vi "GetProbePlanCoordinates.vi"(8 "Use index as X coord":bool=TRUE, 9 "Probe Card Channels":i32=1) -> (0 "file path":string, 2 "OK?":bool, 3 "Array":T1(array[cluster]))   [LabVIEW 2018] (continued)
  out "String":string="There\tmust\tbe\tat\tleast\tone\tregion\nRegion=Segment\t3T\nLabel=Strip\t1\tX=-1082.31\ty=-40425.51 \nLabel=Strip\t2\tX=-725.71\ty=-40380.45 \nLabel=Strip\t3\tX=-1066.76\ty=-40277.87 \nLabel=Strip\t4\tX=-710.17\ty=-40232.68 \nLabel=Strip\t5\tX=-1051.26\ty=-40130.23 \nLabel=Strip\t6\tX=-694.70\ty=-40084.90 \nLabel=Strip\t7\tX=-1035.82\ty=-39982.58 \nLabel=Strip\t8\tX=-679.28\ty=-39937.11 \nLabel=Strip\t9\tX=-1020.44\ty=-39834.92 \nLabel=Strip\t10\tX=-663.91\ty=-39789.32 \nLabel=Strip\t11\tX=-1005.12\ty=-39687.26 \nLabel=Strip\t12\tX=-648.61\ty=-39641.51 \nLabel=Strip\t13\tX=-989.85\ty=-39539.59 \nLabel=Strip\t14\tX=-633.36\ty=-39493.70 \nLabel=Strip\t15\tX=-974.64\ty=-39391.91 \nLabel=Strip\t16\tX=-618.16\ty=-39345.89 \nLabel=Strip\t17\tX=-959.49\ty=-39244.23 \nLabel=Strip\t18\tX=-603.03\ty=-39198.06 \nLabel=Strip\t19\tX=-944.39\ty=-39096.54 \nLabel=Strip\t20\tX=-587.95\ty=-39050.23 \nLabel=Strip\t21\tX=-929.35\ty=-38948.84 \nLabel=Strip\t22\tX=-572.93\ty=-38902.40 \nLabel=Strip\t23\tX=-914.37\ty=-38801.13 \nLabel=Strip\t24\tX=-557.96\ty=-38754.55 \nLabel=Strip\t25\tX=-899.44\ty=-38653.42 \nLabel=Strip\t26\tX=-543.05\ty=-38606.70 \nLabel=Strip\t27\tX=-884.57\ty=-38505.70 \nLabel=Strip\t28\tX=-528.20\ty=-38458.84 \nLabel=Strip\t29\tX=-869.76\ty=-38357.97 \nLabel=Strip\t30\tX=-513.41\ty=-38310.98 \nLabel=Strip\t31\tX=-855.00\ty=-38210.23 \nLabel=Strip\t32\tX=-498.67\ty=-38163.10 \nLabel=Strip\t33\tX=-840.30\ty=-38062.49 \nLabel=Strip\t34\tX=-483.98\ty=-38015.22 \nLabel=Strip\t35\tX=-825.66\ty=-37914.74 \nLabel=Strip\t36\tX=-469.36\ty=-37867.34 \nLabel=Strip\t37\tX=-811.07\ty=-37766.99 \nLabel=Strip\t38\tX=-454.79\ty=-37719.44 \nLabel=Strip\t39\tX=-796.54\ty=-37619.23 \nLabel=Strip\t40\tX=-440.28\ty=-37571.54 \nLabel=Strip\t41\tX=-782.07\ty=-37471.46 \nLabel=Strip\t42\tX=-425.83\ty=-37423.64 \nLabel=Strip\t43\tX=-767.66\ty=-37323.68 \nLabel=Strip\t44\tX=-411.43\ty=-37275.72 \nLabel=Strip\t45\tX=-753.30\ty=-37175.90 \nLabel=Strip\t46\tX=-397.09\ty=-37127.80 \nLabel=Strip\t47\tX=-739.00\ty=-37028.11 \nLabel=Strip\t48\tX=-382.81\ty=-36979.87 \nLabel=Strip\t49\tX=-724.75\ty=-36880.31 \nLabel=Strip\t50\tX=-368.58\ty=-36831.94 \nLabel=Strip\t51\tX=-710.56\ty=-36732.51 \nLabel=Strip\t52\tX=-354.41\ty=-36684.00 \nLabel=Strip\t53\tX=-696.43\ty=-36584.70 \nLabel=Strip\t54\tX=-340.30\ty=-36536.05 \nLabel=Strip\t55\tX=-682.36\ty=-36436.88 \nLabel=Strip\t56\tX=-326.25\ty=-36388.09 \nLabel=Strip\t57\tX=-668.34\ty=-36289.06 \nLabel=Strip\t58\tX=-312.25\ty=-36240.13 \nLabel=Strip\t59\tX=-654.38\ty=-36141.23 \nLabel=Strip\t60\tX=-298.30\ty=-36092.16 \nLabel=Strip\t61\tX=-640.48\ty=-35993.39 \nLabel=Strip\t62\tX=-284.42\ty=-35944.19 \nLabel=Strip\t63\tX=-626.63\ty=-35845.55 \nLabel=Strip\t64\tX=-270.59\ty=-35796.21 \nLabel=Strip\t65\tX=-612.84\ty=-35697.70 \nLabel=Strip\t66\tX=-256.82\ty=-35648.22 \nLabel=Strip\t67\tX=-599.11\ty=-35549.84 \nLabel=Strip\t68\tX=-243.11\ty=-35500.22 \nLabel=Strip\t69\tX=-585.43\ty=-35401.98 \nLabel=Strip\t70\tX=-229.45\ty=-35352.22 \nLabel=Strip\t71\tX=-571.81\ty=-35254.11 \nLabel=Strip\t72\tX=-215.85\ty=-35204.22 \nLabel=Strip\t73\tX=-558.25\ty=-35106.23 \nLabel=Strip\t74\tX=-202.31\ty=-35056.20 \nLabel=Strip\t75\tX=-544.74\ty=-34958.35 \nLabel=Strip\t76\tX=-188.82\ty=-34908.18 \nLabel=Strip\t77\tX=-531.29\ty=-34810.46 \nLabel=Strip\t78\tX=-175.39\ty=-34760.15 \nLabel=Strip\t79\tX=-517.90\ty=-34662.57 \nLabel=Strip\t80\tX=-162.02\ty=-34612.12 \nLabel=Strip\t81\tX=-504.57\ty=-34514.66 \nLabel=Strip\t82\tX=-148.70\ty=-34464.08 \nLabel=Strip\t83\tX=-491.29\ty=-34366.75 \nLabel=Strip\t84\tX=-135.44\ty=-34316.03 \nLabel=Strip\t85\tX=-478.07\ty=-34218.84 \nLabel=Strip\t86\tX=-122.24\ty=-34167.98 \nLabel=Strip\t87\tX=-464.90\ty=-34070.92 \nLabel=Strip\t88\tX=-109.10\ty=-34019.92 \nLabel=Strip\t89\tX=-451.80\ty=-33922.99 \nLabel=Strip\t90\tX=-96.01\ty=-33871.85 \nLabel=Strip\t91\tX=-438.75\ty=-33775.06 \nLabel=Strip\t92\tX=-82.98\ty=-33723.78 \nLabel=Strip\t93\tX=-425.75\ty=-33627.12 \nLabel=Strip\t94\tX=-70.01\ty=-33575.70 \nLabel=Strip\t95\tX=-412.82\ty=-33479.17 \nLabel=Strip\t96\tX=-57.09\ty=-33427.62 \nLabel=Strip\t97\tX=-399.94\ty=-33331.21 \nLabel=Strip\t98\tX=-44.23\ty=-33279.53 \nLabel=Strip\t99\tX=-387.12\ty=-33183.26 \nLabel=Strip\t100\tX=-31.43\ty=-33131.43 \nLabel=Strip\t101\tX=-374.35\ty=-33035.29 \nLabel=Strip\t102\tX=-18.68\ty=-32983.32 \nLabel=Strip\t103\tX=-361.64\ty=-32887.32 \nLabel=Strip\t104\tX=-5.99\ty=-32835.22 \nLabel=Strip\t105\tX=-348.99\ty=-32739.34 \nLabel=Strip\t106\tX=6.64\ty=-32687.10 \nLabel=Strip\t107\tX=-336.40\ty=-32591.36 \nLabel=Strip\t108\tX=19.21\ty=-32538.98 \nLabel=Strip\t109\tX=-323.86\ty=-32443.37 \nLabel=Strip\t110\tX=31.73\ty=-32390.85 \nLabel=Strip\t111\tX=-311.38\ty=-32295.37 \nLabel=Strip\t112\tX=44.19\ty=-32242.71 \nLabel=Strip\t113\tX=-298.95\ty=-32147.37 \nLabel=Strip\t114\tX=56.59\ty=-32094.57 \nLabel=Strip\t115\tX=-286.59\ty=-31999.36 \nLabel=Strip\t116\tX=68.94\ty=-31946.43 \nLabel=Strip\t117\tX=-274.28\ty=-31851.34 \nLabel=Strip\t118\tX=81.23\ty=-31798.27 \nLabel=Strip\t119\tX=-262.02\ty=-31703.32 \nLabel=Strip\t120\tX=93.46\ty=-31650.12 \nLabel=Strip\t121\tX=-249.83\ty=-31555.30 \nLabel=Strip\t122\tX=105.64\ty=-31501.95 \nLabel=Strip\t123\tX=-237.69\ty=-31407.26 \nLabel=Strip\t124\tX=117.76\ty=-31353.78 \nLabel=Strip\t125\tX=-225.61\ty=-31259.22 \nLabel=Strip\t126\tX=129.82\ty=-31205.60 \nLabel=Strip\t127\tX=-213.58\ty=-31111.18 \nLabel=Strip\t128\tX=141.82\ty=-31057.42 \nLabel=Strip\t129\tX=-201.61\ty=-30963.13 \nLabel=Strip\t130\tX=153.77\ty=-30909.23 \nLabel=Strip\t131\tX=-189.70\ty=-30815.07 \nLabel=Strip\t132\tX=165.66\ty=-30761.04 \nLabel=Strip\t133\tX=-177.85\ty=-30667.01 \nLabel=Strip\t134\tX=177.49\ty=-30612.84 \nLabel=Strip\t135\tX=-166.05\ty=-30518.94 \nLabel=Strip\t136\tX=189.27\ty=-30464.63 \nLabel=Strip\t137\tX=-154.31\ty=-30370.87 \nLabel=Strip\t138\tX=200.99\ty=-30316.42 \nLabel=Strip\t139\tX=-142.63\ty=-30222.79 \nLabel=Strip\t140\tX=212.65\ty=-30168.20 \nLabel=Strip\t141\tX=-131.00\ty=-30074.70 \nLabel=Strip\t142\tX=224.26\ty=-30019.98 \nLabel=Strip\t143\tX=-119.43\ty=-29926.61 \nLabel=Strip\t144\tX=235.81\ty=-29871.75 \nLabel=Strip\t145\tX=-107.92\ty=-29778.51 \nLabel=Strip\t146\tX=247.30\ty=-29723.52 \nLabel=Strip\t147\tX=-96.46\ty=-29630.41 \nLabel=Strip\t148\tX=258.73\ty=-29575.27 \nLabel=Strip\t149\tX=-85.07\ty=-29482.30 \nLabel=Strip\t150\tX=270.11\ty=-29427.03 \nLabel=Strip\t151\tX=-73.72\ty=-29334.19 \nLabel=Strip\t152\tX=281.43\ty=-29278.78 \nLabel=Strip\t153\tX=-62.44\ty=-29186.07 \nLabel=Strip\t154\tX=292.69\ty=-29130.52 \nLabel=Strip\t155\tX=-51.21\ty=-29037.94 \nLabel=Strip\t156\tX=303.90\ty=-28982.25 \nLabel=Strip\t157\tX=-40.04\ty=-28889.81 \nLabel=Strip\t158\tX=315.04\ty=-28833.99 \nLabel=Strip\t159\tX=-28.93\ty=-28741.67 \nLabel=Strip\t160\tX=326.14\ty=-28685.71 \nLabel=Strip\t161\tX=-17.87\ty=-28593.53 \nLabel=Strip\t162\tX=337.17\ty=-28537.43 \nLabel=Strip\t163\tX=-6.87\ty=-28445.38 \nLabel=Strip\t164\tX=348.15\ty=-28389.14 \nLabel=Strip\t165\tX=4.07\ty=-28297.23 \nLabel=Strip\t166\tX=359.07\ty=-28240.85 \nLabel=Strip\t167\tX=14.95\ty=-28149.07 \nLabel=Strip\t168\tX=369.93\ty=-28092.56 \nLabel=Strip\t169\tX=25.78\ty=-28000.91 \nLabel=Strip\t170\tX=380.74\ty=-27944.25 \nLabel=Strip\t171\tX=36.55\ty=-27852.74 \nLabel=Strip\t172\tX=391.49\ty=-27795.95 \nLabel=Strip\t173\tX=47.26\ty=-27704.56 \nLabel=Strip\t174\tX=402.18\ty=-27647.63 \nLabel=Strip\t175\tX=57.92\ty=-27556.38 \nLabel=Strip\t176\tX=412.81\ty=-27499.32 \nLabel=Strip\t177\tX=68.52\ty=-27408.19 \nLabel=Strip\t178\tX=423.39\ty=-27350.99 \nLabel=Strip\t179\tX=79.06\ty=-27260.00 \nLabel=Strip\t180\tX=433.91\ty=-27202.66 \nLabel=Strip\t181\tX=89.55\ty=-27111.81 \nLabel=Strip\t182\tX=444.37\ty=-27054.33 \nLabel=Strip\t183\tX=99.98\ty=-26963.60 \nLabel=Strip\t184\tX=454.78\ty=-26905.99 \nLabel=Strip\t185\tX=110.35\ty=-26815.40 \nLabel=Strip\t186\tX=465.13\ty=-26757.64 \nLabel=Strip\t187\tX=120.66\ty=-26667.18 \nLabel=Strip\t188\tX=475.42\ty=-26609.29 \nLabel=Strip\t189\tX=130.92\ty=-26518.96 \nLabel=Strip\t190\tX=485.66\ty=-26460.93 \nLabel=Strip\t191\tX=141.12\ty=-26370.74 \nLabel=Strip\t192\tX=495.83\ty=-26312.57 \nLabel=Strip\t193\tX=151.26\ty=-26222.51 \nLabel=Strip\t194\tX=505.96\ty=-26164.21 \nLabel=Strip\t195\tX=161.35\ty=-26074.28 \nLabel=Strip\t196\tX=516.02\ty=-26015.84 \nLabel=Strip\t197\tX=171.38\ty=-25926.04 \nLabel=Strip\t198\tX=526.02\ty=-25867.46 \nLabel=Strip\t199\tX=181.35\ty=-25777.80 \nLabel=Strip\t200\tX=535.97\ty=-25719.08 \nLabel=Strip\t201\tX=191.26\ty=-25629.55 \nLabel=Strip\t202\tX=545.87\ty=-25570.69 \nLabel=Strip\t203\tX=201.12\ty=-25481.29 \nLabel=Strip\t204\tX=555.70\ty=-25422.30 \nLabel=Strip\t205\tX=210.92\ty=-25333.03 \nLabel=Strip\t206\tX=565.48\ty=-25273.90 \nLabel=Strip\t207\tX=220.66\ty=-25184.77 \nLabel=Strip\t208\tX=575.20\ty=-25125.50 \nLabel=Strip\t209\tX=230.35\ty=-25036.50 \nLabel=Strip\t210\tX=584.86\ty=-24977.09 \nLabel=Strip\t211\tX=239.98\ty=-24888.22 \nLabel=Strip\t212\tX=594.47\ty=-24828.68 \nLabel=Strip\t213\tX=249.55\ty=-24739.94 \nLabel=Strip\t214\tX=604.02\ty=-24680.26 \nLabel=Strip\t215\tX=259.07\ty=-24591.66 \nLabel=Strip\t216\tX=613.51\ty=-24531.84 \nLabel=Strip\t217\tX=268.53\ty=-24443.37 \nLabel=Strip\t218\tX=622.94\ty=-24383.41 \nLabel=Strip\t219\tX=277.93\ty=-24295.07 \nLabel=Strip\t220\tX=632.32\ty=-24234.98 \nLabel=Strip\t221\tX=287.27\ty=-24146.77 \nLabel=Strip\t222\tX=641.64\ty=-24086.54 \nLabel=Strip\t223\tX=296.56\ty=-23998.47 \nLabel=Strip\t224\tX=650.91\ty=-23938.10 \nLabel=Strip\t225\tX=305.78\ty=-23850.16 \nLabel=Strip\t226\tX=660.11\ty=-23789.65 \nLabel=Strip\t227\tX=314.96\ty=-23701.85 \nLabel=Strip\t228\tX=669.26\ty=-23641.20 \nLabel=Strip\t229\tX=324.07\ty=-23553.53 \nLabel=Strip\t230\tX=678.35\ty=-23492.75 \nLabel=Strip\t231\tX=333.13\ty=-23405.20 \nLabel=Strip\t232\tX=687.39\ty=-23344.29 \nLabel=Strip\t233\tX=342.13\ty=-23256.88 \nLabel=Strip\t234\tX=696.36\ty=-23195.82 \nLabel=Strip\t235\tX=351.07\ty=-23108.54 \nLabel=Strip\t236\tX=705.28\ty=-23047.35 \nLabel=Strip\t237\tX=359.96\ty=-22960.20 \nLabel=Strip\t238\tX=714.15\ty=-22898.87 \nLabel=Strip\t239\tX=368.79\ty=-22811.86 \nLabel=Strip\t240\tX=722.95\ty=-22750.39 \nLabel=Strip\t241\tX=377.56\ty=-22663.51 \nLabel=Strip\t242\tX=731.70\ty=-22601.91 \nLabel=Strip\t243\tX=386.28\ty=-22515.16 \nLabel=Strip\t244\tX=740.39\ty=-22453.42 \nLabel=Strip\t245\tX=394.94\ty=-22366.80 \nLabel=Strip\t246\tX=749.03\ty=-22304.92 \nLabel=Strip\t247\tX=403.54\ty=-22218.44 \nLabel=Strip\t248\tX=757.60\ty=-22156.40 \nLabel=Strip\t249\tX=412.08\ty=-22070.08 \nLabel=Strip\t250\tX=766.12\ty=-22007.92 \nLabel=Strip\t251\tX=420.57\ty=-21921.71 \nLabel=Strip\t252\tX=774.58\ty=-21859.41 \nLabel=Strip\t253\tX=428.99\ty=-21773.33 \nLabel=Strip\t254\tX=782.99\ty=-21710.90 \nLabel=Strip\t255\tX=437.37\ty=-21624.95 \nLabel=Strip\t256\tX=791.34\ty=-21562.38 \nLabel=Strip\t257\tX=445.68\ty=-21476.57 \nLabel=Strip\t258\tX=799.63\ty=-21413.86 \nLabel=Strip\t259\tX=453.94\ty=-21328.18 \nLabel=Strip\t260\tX=807.86\ty=-21265.34 \nLabel=Strip\t261\tX=462.14\ty=-21179.78 \nLabel=Strip\t262\tX=816.04\ty=-21116.81 \nLabel=Strip\t263\tX=470.28\ty=-21031.39 \nLabel=Strip\t264\tX=824.16\ty=-20968.27 \nLabel=Strip\t265\tX=478.37\ty=-20882.98 \nLabel=Strip\t266\tX=832.22\ty=-20819.73 \nLabel=Strip\t267\tX=486.40\ty=-20734.58 \nLabel=Strip\t268\tX=840.22\ty=-20671.19 \nLabel=Strip\t269\tX=494.37\ty=-20586.17 \nLabel=Strip\t270\tX=848.17\ty=-20522.64 \nLabel=Strip\t271\tX=502.28\ty=-20437.75 \nLabel=Strip\t272\tX=856.06\ty=-20374.08 \nLabel=Strip\t273\tX=510.14\ty=-20289.33 \nLabel=Strip\t274\tX=863.89\ty=-20225.53 \nLabel=Strip\t275\tX=517.94\ty=-20140.91 \nLabel=Strip\t276\tX=871.67\ty=-20076.97 \nLabel=Strip\t277\tX=525.68\ty=-19992.48 \nLabel=Strip\t278\tX=879.39\ty=-19928.40 \nLabel=Strip\t279\tX=533.37\ty=-19844.05 \nLabel=Strip\t280\tX=887.05\ty=-19779.83 \nLabel=Strip\t281\tX=541.00\ty=-19695.61 \nLabel=Strip\t282\tX=894.65\ty=-19631.26 \nLabel=Strip\t283\tX=548.57\ty=-19547.17 \nLabel=Strip\t284\tX=902.20\ty=-19482.68 \nLabel=Strip\t285\tX=556.08\ty=-19398.72 \nLabel=Strip\t286\tX=909.69\ty=-19334.10 \nLabel=Strip\t287\tX=563.54\ty=-19250.27 \nLabel=Strip\t288\tX=917.12\ty=-19185.51 \nLabel=Strip\t289\tX=570.94\ty=-19101.82 \nLabel=Strip\t290\tX=924.49\ty=-19036.92 \nLabel=Strip\t291\tX=578.28\ty=-18953.36 \nLabel=Strip\t292\tX=931.81\ty=-18888.32 \nLabel=Strip\t293\tX=585.57\ty=-18804.90 \nLabel=Strip\t294\tX=939.07\ty=-18739.72 \nLabel=Strip\t295\tX=592.80\ty=-18656.43 \nLabel=Strip\t296\tX=946.27\ty=-18591.12 \nLabel=Strip\t297\tX=599.97\ty=-18507.96 \nLabel=Strip\t298\tX=953.42\ty=-18442.51 \nLabel=Strip\t299\tX=607.08\ty=-18359.49 \nLabel=Strip\t300\tX=960.51\ty=-18293.90 \nLabel=Strip\t301\tX=614.14\ty=-18211.01 \nLabel=Strip\t302\tX=967.54\ty=-18145.29 \nLabel=Strip\t303\tX=621.14\ty=-18062.53 \nLabel=Strip\t304\tX=974.51\ty=-17996.67 \nLabel=Strip\t305\tX=628.08\ty=-17914.04 \nLabel=Strip\t306\tX=981.43\ty=-17848.04 \nLabel=Strip\t307\tX=634.96\ty=-17765.55 \nLabel=Strip\t308\tX=988.29\ty=-17699.42 \nLabel=Strip\t309\tX=641.79\ty=-17617.06 \nLabel=Strip\t310\tX=995.09\ty=-17550.78 \nLabel=Strip\t311\tX=648.56\ty=-17468.56 \nLabel=Strip\t312\tX=1001.84\ty=-17402.15 \nLabel=Strip\t313\tX=655.27\ty=-17320.06 \nLabel=Strip\t314\tX=1008.52\ty=-17253.51 \nLabel=Strip\t315\tX=661.93\ty=-17171.55 \nLabel=Strip\t316\tX=1015.15\ty=-17104.87 \nLabel=Strip\t317\tX=668.53\ty=-17023.04 \nLabel=Strip\t318\tX=1021.72\ty=-16956.22 \nLabel=Strip\t319\tX=675.07\ty=-16874.53 \nLabel=Strip\t320\tX=1028.24\ty=-16807.57 \nLabel=Strip\t321\tX=681.55\ty=-16726.01 \nLabel=Strip\t322\tX=1034.70\ty=-16658.91 \nLabel=Strip\t323\tX=687.98\ty=-16577.49 \nLabel=Strip\t324\tX=1041.10\ty=-16510.26 \nLabel=Strip\t325\tX=694.35\ty=-16428.96 \nLabel=Strip\t326\tX=1047.44\ty=-16361.59 \nLabel=Strip\t327\tX=700.66\ty=-16280.43 \nLabel=Strip\t328\tX=1053.73\ty=-16212.93 \nLabel=Strip\t329\tX=706.91\ty=-16131.90 \nLabel=Strip\t330\tX=1059.96\ty=-16064.26 \nLabel=Strip\t331\tX=713.11\ty=-15983.36 \nLabel=Strip\t332\tX=1066.13\ty=-15915.59 \nLabel=Strip\t333\tX=719.25\ty=-15834.82 \nLabel=Strip\t334\tX=1072.24\ty=-15766.91 \nLabel=Strip\t335\tX=725.33\ty=-15686.28 \nLabel=Strip\t336\tX=1078.30\ty=-15618.23 \nLabel=Strip\t337\tX=731.36\ty=-15537.73 \nLabel=Strip\t338\tX=1084.30\ty=-15469.54 \nLabel=Strip\t339\tX=737.33\ty=-15389.18 \nLabel=Strip\t340\tX=1090.24\ty=-15320.86 \nLabel=Strip\t341\tX=743.24\ty=-15240.63 \nLabel=Strip\t342\tX=1096.13\ty=-15172.16 \nLabel=Strip\t343\tX=749.09\ty=-15092.07 \nLabel=Strip\t344\tX=1101.95\ty=-15023.47 \nLabel=Strip\t345\tX=754.89\ty=-14943.51 \nLabel=Strip\t346\tX=1107.72\ty=-14874.77 \nLabel=Strip\t347\tX=760.63\ty=-14794.94 \nLabel=Strip\t348\tX=1113.44\ty=-14726.07 \nLabel=Strip\t349\tX=766.31\ty=-14646.37 \nLabel=Strip\t350\tX=1119.09\ty=-14577.36 \nLabel=Strip\t351\tX=771.93\ty=-14497.80 \nLabel=Strip\t352\tX=1124.69\ty=-14428.65 \nLabel=Strip\t353\tX=777.50\ty=-14349.23 \nLabel=Strip\t354\tX=1130.23\ty=-14279.94 \nLabel=Strip\t355\tX=783.01\ty=-14200.65 \nLabel=Strip\t356\tX=1135.71\ty=-14131.23 \nLabel=Strip\t357\tX=788.47\ty=-14052.07 \nLabel=Strip\t358\tX=1141.14\ty=-13982.51 \nLabel=Strip\t359\tX=793.86\ty=-13903.48 \nLabel=Strip\t360\tX=1146.51\ty=-13833.78 \nLabel=Strip\t361\tX=799.20\ty=-13754.89 \nLabel=Strip\t362\tX=1151.82\ty=-13685.06 \nLabel=Strip\t363\tX=804.48\ty=-13606.30 \nLabel=Strip\t364\tX=1157.07\ty=-13536.33 \nLabel=Strip\t365\tX=809.70\ty=-13457.70 \nLabel=Strip\t366\tX=1162.27\ty=-13387.59 \nLabel=Strip\t367\tX=814.87\ty=-13309.10 \nLabel=Strip\t368\tX=1167.41\ty=-13238.86 \nLabel=Strip\t369\tX=819.98\ty=-13160.50 \nLabel=Strip\t370\tX=1172.49\ty=-13090.12 \nLabel=Strip\t371\tX=825.03\ty=-13011.89 \nLabel=Strip\t372\tX=1177.51\ty=-12941.38 \nLabel=Strip\t373\tX=830.02\ty=-12863.28 \nLabel=Strip\t374\tX=1182.48\ty=-12792.63 \nLabel=Strip\t375\tX=834.96\ty=-12714.67 \nLabel=Strip\t376\tX=1187.39\ty=-12643.88 \nLabel=Strip\t377\tX=839.84\ty=-12566.06 \nLabel=Strip\t378\tX=1192.24\ty=-12495.13 \nLabel=Strip\t379\tX=844.66\ty=-12417.44 \nLabel=Strip\t380\tX=1197.04\ty=-12346.37 \nLabel=Strip\t381\tX=849.43\ty=-12268.82 \nLabel=Strip\t382\tX=1201.77\ty=-12197.62 \nLabel=Strip\t383\tX=854.13\ty=-12120.19 \nLabel=Strip\t384\tX=1206.45\ty=-12048.85 \nLabel=Strip\t385\tX=858.79\ty=-11971.56 \nLabel=Strip\t386\tX=1211.08\ty=-11900.09 \nLabel=Strip\t387\tX=863.38\ty=-11822.93 \nLabel=Strip\t388\tX=1215.64\ty=-11751.32 \nLabel=Strip\t389\tX=867.91\ty=-11674.30 \nLabel=Strip\t390\tX=1220.15\ty=-11602.55 \nLabel=Strip\t391\tX=872.39\ty=-11525.66 \nLabel=Strip\t392\tX=1224.60\ty=-11453.78 \nLabel=Strip\t393\tX=876.81\ty=-11377.02 \nLabel=Strip\t394\tX=1228.99\ty=-11305.00 \nLabel=Strip\t395\tX=881.18\ty=-11228.38 \nLabel=Strip\t396\tX=1233.33\ty=-11156.22 \nLabel=Strip\t397\tX=885.48\ty=-11079.73 \nLabel=Strip\t398\tX=1237.61\ty=-11007.44 \nLabel=Strip\t399\tX=889.73\ty=-10931.08 \nLabel=Strip\t400\tX=1241.83\ty=-10858.65 \nLabel=Strip\t401\tX=893.92\ty=-10782.43 \nLabel=Strip\t402\tX=1245.99\ty=-10709.86 \nLabel=Strip\t403\tX=898.06\ty=-10633.77 \nLabel=Strip\t404\tX=1250.10\ty=-10561.07 \nLabel=Strip\t405\tX=902.14\ty=-10484.45 \nLabel=Strip\t406\tX=1254.15\ty=-10411.48 \nLabel=Strip\t407\tX=906.15\ty=-10336.06 \nLabel=Strip\t408\tX=1258.14\ty=-10263.09 \nLabel=Strip\t409\tX=910.12\ty=-10187.67 \nLabel=Strip\t410\tX=1262.07\ty=-10114.69 \nLabel=Strip\t411\tX=914.02\ty=-10039.27 \nLabel=Strip\t412\tX=1265.95\ty=-9966.29 \nLabel=Strip\t413\tX=917.87\ty=-9890.87 \nLabel=Strip\t414\tX=1269.77\ty=-9817.89 \nLabel=Strip\t415\tX=921.66\ty=-9742.46 \nLabel=Strip\t416\tX=1273.53\ty=-9668.26 \nLabel=Strip\t417\tX=925.39\ty=-9593.11 \nLabel=Strip\t418\tX=1277.23\ty=-9519.45 \nLabel=Strip\t419\tX=929.06\ty=-9444.43 \nLabel=Strip\t420\tX=1280.88\ty=-9370.63 \nLabel=Strip\t421\tX=932.68\ty=-9295.75 \nLabel=Strip\t422\tX=1284.47\ty=-9221.82 \nLabel=Strip\t423\tX=936.24\ty=-9147.07 \nLabel=Strip\t424\tX=1288.00\ty=-9073.00 \nLabel=Strip\t425\tX=939.75\ty=-8998.38 \nLabel=Strip\t426\tX=1291.48\ty=-8924.17 \nLabel=Strip\t427\tX=943.19\ty=-8849.69 \nLabel=Strip\t428\tX=1294.89\ty=-8775.35 \nLabel=Strip\t429\tX=946.58\ty=-8701.00 \nLabel=Strip\t430\tX=1298.25\ty=-8626.52 \nLabel=Strip\t431\tX=949.91\ty=-8552.31 \nLabel=Strip\t432\tX=1301.55\ty=-8477.69 \nLabel=Strip\t433\tX=953.18\ty=-8403.61 \nLabel=Strip\t434\tX=1304.80\ty=-8328.86 \nLabel=Strip\t435\tX=956.40\ty=-8254.91 \nLabel=Strip\t436\tX=1307.99\ty=-8180.02 \nLabel=Strip\t437\tX=959.56\ty=-8106.21 \nLabel=Strip\t438\tX=1311.12\ty=-8031.19 \nLabel=Strip\t439\tX=962.66\ty=-7957.51 \nLabel=Strip\t440\tX=1314.19\ty=-7882.35 \nLabel=Strip\t441\tX=965.71\ty=-7808.80 \nLabel=Strip\t442\tX=1317.20\ty=-7733.50 \nLabel=Strip\t443\tX=968.69\ty=-7660.09 \nLabel=Strip\t444\tX=1320.16\ty=-7584.66 \nLabel=Strip\t445\tX=971.62\ty=-7511.38 \nLabel=Strip\t446\tX=1323.06\ty=-7435.81 \nLabel=Strip\t447\tX=974.49\ty=-7362.67 \nLabel=Strip\t448\tX=1325.90\ty=-7286.96 \nLabel=Strip\t449\tX=977.31\ty=-7213.95 \nLabel=Strip\t450\tX=1328.69\ty=-7138.11 \nLabel=Strip\t451\tX=980.06\ty=-7065.23 \nLabel=Strip\t452\tX=1331.42\ty=-6989.25 \nLabel=Strip\t453\tX=982.76\ty=-6916.51 \nLabel=Strip\t454\tX=1334.09\ty=-6840.40 \nLabel=Strip\t455\tX=985.41\ty=-6767.79 \nLabel=Strip\t456\tX=1336.70\ty=-6691.54 \nLabel=Strip\t457\tX=987.99\ty=-6619.06 \nLabel=Strip\t458\tX=1339.26\ty=-6542.67 \nLabel=Strip\t459\tX=990.52\ty=-6470.33 \nLabel=Strip\t460\tX=1341.75\ty=-6393.81 \nLabel=Strip\t461\tX=992.99\ty=-6321.60 \nLabel=Strip\t462\tX=1344.19\ty=-6244.94 \nLabel=Strip\t463\tX=995.40\ty=-6172.87 \nLabel=Strip\t464\tX=1346.58\ty=-6096.07 \nLabel=Strip\t465\tX=997.76\ty=-6024.14 \nLabel=Strip\t466\tX=1348.90\ty=-5947.20 \nLabel=Strip\t467\tX=1000.05\ty=-5875.40 \nLabel=Strip\t468\tX=1351.17\ty=-5798.33 \nLabel=Strip\t469\tX=1002.29\ty=-5726.66 \nLabel=Strip\t470\tX=1353.38\ty=-5649.46 \nLabel=Strip\t471\tX=1004.48\ty=-5577.92 \nLabel=Strip\t472\tX=1355.53\ty=-5500.58 \nLabel=Strip\t473\tX=1006.60\ty=-5429.18 \nLabel=Strip\t474\tX=1357.63\ty=-5351.70 \nLabel=Strip\t475\tX=1008.67\ty=-5280.43 \nLabel=Strip\t476\tX=1359.67\ty=-5202.82 \nLabel=Strip\t477\tX=1010.68\ty=-5131.68 \nLabel=Strip\t478\tX=1361.65\ty=-5053.93 \nLabel=Strip\t479\tX=1012.63\ty=-4982.93 \nLabel=Strip\t480\tX=1363.57\ty=-4905.05 \nLabel=Strip\t481\tX=1014.53\ty=-4834.18 \nLabel=Strip\t482\tX=1365.44\ty=-4756.16 \nLabel=Strip\t483\tX=1016.37\ty=-4685.43 \nLabel=Strip\t484\tX=1367.25\ty=-4607.27 \nLabel=Strip\t485\tX=1018.15\ty=-4536.67 \nLabel=Strip\t486\tX=1369.00\ty=-4458.38 \nLabel=Strip\t487\tX=1019.87\ty=-4387.92 \nLabel=Strip\t488\tX=1370.69\ty=-4309.48 \nLabel=Strip\t489\tX=1021.54\ty=-4239.16 \nLabel=Strip\t490\tX=1372.32\ty=-4160.59 \nLabel=Strip\t491\tX=1023.15\ty=-4090.40 \nLabel=Strip\t492\tX=1373.90\ty=-4011.69 \nLabel=Strip\t493\tX=1024.70\ty=-3941.63 \nLabel=Strip\t494\tX=1375.42\ty=-3862.79 \nLabel=Strip\t495\tX=1026.19\ty=-3792.87 \nLabel=Strip\t496\tX=1376.89\ty=-3713.89 \nLabel=Strip\t497\tX=1027.63\ty=-3644.10 \nLabel=Strip\t498\tX=1378.29\ty=-3564.99 \nLabel=Strip\t499\tX=1029.01\ty=-3495.33 \nLabel=Strip\t500\tX=1379.64\ty=-3416.08 \nLabel=Strip\t501\tX=1030.33\ty=-3346.56 \nLabel=Strip\t502\tX=1380.93\ty=-3267.18 \nLabel=Strip\t503\tX=1031.59\ty=-3197.79 \nLabel=Strip\t504\tX=1382.16\ty=-3118.27 \nLabel=Strip\t505\tX=1032.80\ty=-3049.01 \nLabel=Strip\t506\tX=1383.34\ty=-2969.36 \nLabel=Strip\t507\tX=1033.95\ty=-2900.24 \nLabel=Strip\t508\tX=1384.46\ty=-2820.44 \nLabel=Strip\t509\tX=1035.04\ty=-2751.46 \nLabel=Strip\t510\tX=1385.52\ty=-2671.53 \nLabel=Strip\t511\tX=1036.07\ty=-2602.68 \nLabel=Strip\t512\tX=1386.52\ty=-2522.61 \nLabel=Strip\t513\tX=1037.05\ty=-2453.90 \nLabel=Strip\t514\tX=1387.47\ty=-2373.70 \nLabel=Strip\t515\tX=1037.97\ty=-2305.11 \nLabel=Strip\t516\tX=1388.36\ty=-2224.78 \nLabel=Strip\t517\tX=1038.83\ty=-2156.33 \nLabel=Strip\t518\tX=1389.19\ty=-2075.86 \nLabel=Strip\t519\tX=1039.63\ty=-2007.54 \nLabel=Strip\t520\tX=1389.96\ty=-1926.94 \nLabel=Strip\t521\tX=1040.38\ty=-1858.75 \nLabel=Strip\t522\tX=1390.68\ty=-1778.01 \nLabel=Strip\t523\tX=1041.07\ty=-1709.96 \nLabel=Strip\t524\tX=1391.33\ty=-1629.09 \nLabel=Strip\t525\tX=1041.70\ty=-1561.17 \nLabel=Strip\t526\tX=1391.93\ty=-1480.16 \nLabel=Strip\t527\tX=1042.28\ty=-1412.38 \nLabel=Strip\t528\tX=1392.48\ty=-1331.23 \nLabel=Strip\t529\tX=1042.79\ty=-1263.59 \nLabel=Strip\t530\tX=1392.96\ty=-1182.30 \nLabel=Strip\t531\tX=1043.25\ty=-1114.79 \nLabel=Strip\t532\tX=1393.39\ty=-1033.37 \nLabel=Strip\t533\tX=1043.65\ty=-965.99 \nLabel=Strip\t534\tX=1393.76\ty=-884.44 \nLabel=Strip\t535\tX=1044.00\ty=-817.20 \nLabel=Strip\t536\tX=1394.07\ty=-735.50 \nLabel=Strip\t537\tX=1044.29\ty=-668.40 \nLabel=Strip\t538\tX=1394.33\ty=-586.57 \nLabel=Strip\t539\tX=1044.52\ty=-519.59 \nLabel=Strip\t540\tX=1394.53\ty=-437.63 \nLabel=Strip\t541\tX=1044.69\ty=-370.79 \nLabel=Strip\t542\tX=1394.67\ty=-288.69 \nLabel=Strip\t543\tX=1044.80\ty=-221.99 \nLabel=Strip\t544\tX=1394.75\ty=-139.75 \nLabel=Strip\t545\tX=1044.86\ty=-73.18 \nLabel=Strip\t546\tX=1394.78\ty=9.19 \nLabel=Strip\t547\tX=1044.86\ty=75.62 \nLabel=Strip\t548\tX=1394.74\ty=158.14 \nLabel=Strip\t549\tX=1044.80\ty=224.43 \nLabel=Strip\t550\tX=1394.65\ty=307.08 \nLabel=Strip\t551\tX=1044.69\ty=373.24 \nLabel=Strip\t552\tX=1394.51\ty=456.02 \nLabel=Strip\t553\tX=1044.51\ty=522.05 \nLabel=Strip\t554\tX=1394.30\ty=604.97 \nLabel=Strip\t555\tX=1044.28\ty=670.87 \nLabel=Strip\t556\tX=1394.04\ty=753.92 \nLabel=Strip\t557\tX=1044.00\ty=819.68 \nLabel=Strip\t558\tX=1393.72\ty=902.87 \nLabel=Strip\t559\tX=1043.65\ty=968.49 \nLabel=Strip\t560\tX=1393.34\ty=1051.82 \nLabel=Strip\t561\tX=1043.25\ty=1117.31 \nLabel=Strip\t562\tX=1392.91\ty=1200.77 \nLabel=Strip\t563\tX=1042.79\ty=1266.12 \nLabel=Strip\t564\tX=1392.41\ty=1349.72 \nLabel=Strip\t565\tX=1042.27\ty=1414.94 \nLabel=Strip\t566\tX=1391.86\ty=1498.67 \nLabel=Strip\t567\tX=1041.69\ty=1563.76 \nLabel=Strip\t568\tX=1391.26\ty=1647.63 \nLabel=Strip\t569\tX=1041.06\ty=1712.58 \nLabel=Strip\t570\tX=1390.59\ty=1796.58 \nLabel=Strip\t571\tX=1040.37\ty=1861.40 \nLabel=Strip\t572\tX=1389.87\ty=1945.54 \nLabel=Strip\t573\tX=1039.62\ty=2010.22 \nLabel=Strip\t574\tX=1389.09\ty=2094.50 \nLabel=Strip\t575\tX=1038.82\ty=2159.05 \nLabel=Strip\t576\tX=1388.25\ty=2243.46 \nLabel=Strip\t577\tX=1037.95\ty=2307.87 \nLabel=Strip\t578\tX=1387.35\ty=2392.42 \nLabel=Strip\t579\tX=1037.03\ty=2456.70 \nLabel=Strip\t580\tX=1386.40\ty=2541.38 \nLabel=Strip\t581\tX=1036.05\ty=2605.52 \nLabel=Strip\t582\tX=1385.39\ty=2690.34 \nLabel=Strip\t583\tX=1035.02\ty=2754.35 \nLabel=Strip\t584\tX=1384.32\ty=2839.30 \nLabel=Strip\t585\tX=1033.93\ty=2903.18 \nLabel=Strip\t586\tX=1383.20\ty=2988.26 \nLabel=Strip\t587\tX=1032.78\ty=3052.00 \nLabel=Strip\t588\tX=1382.01\ty=3137.23 \nLabel=Strip\t589\tX=1031.57\ty=3200.83 \nLabel=Strip\t590\tX=1380.77\ty=3286.19 \nLabel=Strip\t591\tX=1030.30\ty=3349.66 \nLabel=Strip\t592\tX=1379.47\ty=3435.16 \nLabel=Strip\t593\tX=1028.98\ty=3498.50 \nLabel=Strip\t594\tX=1378.12\ty=3584.12 \nLabel=Strip\t595\tX=1027.60\ty=3647.33 \nLabel=Strip\t596\tX=1376.70\ty=3733.09 \nLabel=Strip\t597\tX=1026.16\ty=3796.16 \nLabel=Strip\t598\tX=1375.23\ty=3882.06 \nLabel=Strip\t599\tX=1024.67\ty=3944.99 \nLabel=Strip\t600\tX=1373.70\ty=4031.03 \nLabel=Strip\t601\tX=1023.11\ty=4093.83 \nLabel=Strip\t602\tX=1372.12\ty=4180.00 \nLabel=Strip\t603\tX=1021.50\ty=4242.66 \nLabel=Strip\t604\tX=1370.47\ty=4328.97 \nLabel=Strip\t605\tX=1019.83\ty=4391.50 \nLabel=Strip\t606\tX=1368.77\ty=4477.94 \nLabel=Strip\t607\tX=1018.11\ty=4540.33 \nLabel=Strip\t608\tX=1367.01\ty=4626.91 \nLabel=Strip\t609\tX=1016.32\ty=4689.17 \nLabel=Strip\t610\tX=1365.20\ty=4775.88 \nLabel=Strip\t611\tX=1014.48\ty=4838.01 \nLabel=Strip\t612\tX=1363.32\ty=4924.86 \nLabel=Strip\t613\tX=1012.59\ty=4986.85 \nLabel=Strip\t614\tX=1361.39\ty=5073.83 \nLabel=Strip\t615\tX=1010.63\ty=5135.68 \nLabel=Strip\t616\tX=1359.40\ty=5222.80 \nLabel=Strip\t617\tX=1008.62\ty=5284.52 \nLabel=Strip\t618\tX=1357.35\ty=5371.78 \nLabel=Strip\t619\tX=1006.55\ty=5433.36 \nLabel=Strip\t620\tX=1355.25\ty=5520.75 \nLabel=Strip\t621\tX=1004.42\ty=5582.20 \nLabel=Strip\t622\tX=1353.09\ty=5669.73 \nLabel=Strip\t623\tX=1002.23\ty=5731.04 \nLabel=Strip\t624\tX=1350.87\ty=5818.70 \nLabel=Strip\t625\tX=999.99\ty=5879.88 \nLabel=Strip\t626\tX=1348.59\ty=5967.68 \nLabel=Strip\t627\tX=997.69\ty=6028.73 \nLabel=Strip\t628\tX=1346.25\ty=6116.66 \nLabel=Strip\t629\tX=995.33\ty=6177.57 \nLabel=Strip\t630\tX=1343.86\ty=6265.63 \nLabel=Strip\t631\tX=992.91\ty=6326.41 \nLabel=Strip\t632\tX=1341.41\ty=6414.61 \nLabel=Strip\t633\tX=990.44\ty=6475.25 \nLabel=Strip\t634\tX=1338.90\ty=6563.59 \nLabel=Strip\t635\tX=987.91\ty=6624.09 \nLabel=Strip\t636\tX=1336.34\ty=6712.57 \nLabel=Strip\t637\tX=985.32\ty=6772.94 \nLabel=Strip\t638\tX=1333.72\ty=6861.54 \nLabel=Strip\t639\tX=982.67\ty=6921.78 \nLabel=Strip\t640\tX=1331.04\ty=7010.52 \nLabel=Strip\t641\tX=979.97\ty=7070.63 \nLabel=Strip\t642\tX=1328.30\ty=7159.50 \nLabel=Strip\t643\tX=977.21\ty=7219.47 \nLabel=Strip\t644\tX=1325.50\ty=7308.48 \nLabel=Strip\t645\tX=974.39\ty=7368.31 \nLabel=Strip\t646\tX=1322.65\ty=7457.46 \nLabel=Strip\t647\tX=971.51\ty=7517.16 \nLabel=Strip\t648\tX=1319.74\ty=7606.44 \nLabel=Strip\t649\tX=968.58\ty=7666.00 \nLabel=Strip\t650\tX=1316.77\ty=7755.42 \nLabel=Strip\t651\tX=965.59\ty=7814.85 \nLabel=Strip\t652\tX=1313.74\ty=7904.40 \nLabel=Strip\t653\tX=962.54\ty=7963.69 \nLabel=Strip\t654\tX=1310.66\ty=8053.38 \nLabel=Strip\t655\tX=959.43\ty=8112.54 \nLabel=Strip\t656\tX=1307.52\ty=8202.36 \nLabel=Strip\t657\tX=956.27\ty=8261.38 \nLabel=Strip\t658\tX=1304.32\ty=8351.34 \nLabel=Strip\t659\tX=953.04\ty=8410.23 \nLabel=Strip\t660\tX=1301.06\ty=8500.32 \nLabel=Strip\t661\tX=949.77\ty=8559.07 \nLabel=Strip\t662\tX=1297.75\ty=8649.30 \nLabel=Strip\t663\tX=946.43\ty=8707.92 \nLabel=Strip\t664\tX=1294.38\ty=8798.28 \nLabel=Strip\t665\tX=943.03\ty=8856.76 \nLabel=Strip\t666\tX=1290.95\ty=8947.26 \nLabel=Strip\t667\tX=939.58\ty=9005.61 \nLabel=Strip\t668\tX=1287.46\ty=9096.24 \nLabel=Strip\t669\tX=936.07\ty=9154.45 \nLabel=Strip\t670\tX=1283.91\ty=9245.22 \nLabel=Strip\t671\tX=932.51\ty=9303.30 \nLabel=Strip\t672\tX=1280.31\ty=9394.20 \nLabel=Strip\t673\tX=928.88\ty=9452.14 \nLabel=Strip\t674\tX=1276.65\ty=9543.18 \nLabel=Strip\t675\tX=925.20\ty=9600.99 \nLabel=Strip\t676\tX=1272.93\ty=9692.16 \nLabel=Strip\t677\tX=921.46\ty=9749.84 \nLabel=Strip\t678\tX=1269.16\ty=9841.14 \nLabel=Strip\t679\tX=917.66\ty=9898.68 \nLabel=Strip\t680\tX=1265.33\ty=9990.12 \nLabel=Strip\t681\tX=913.81\ty=10047.52 \nLabel=Strip\t682\tX=1261.44\ty=10139.10 \nLabel=Strip\t683\tX=909.89\ty=10196.37 \nLabel=Strip\t684\tX=1257.49\ty=10288.08 \nLabel=Strip\t685\tX=905.92\ty=10345.21 \nLabel=Strip\t686\tX=1253.48\ty=10437.06 \nLabel=Strip\t687\tX=901.90\ty=10494.06 \nLabel=Strip\t688\tX=1249.42\ty=10586.04 \nLabel=Strip\t689\tX=897.81\ty=10642.90 \nLabel=Strip\t690\tX=1245.30\ty=10735.02 \nLabel=Strip\t691\tX=893.67\ty=10791.74 \nLabel=Strip\t692\tX=1241.12\ty=10884.00 \nLabel=Strip\t693\tX=889.47\ty=10940.59 \nLabel=Strip\t694\tX=1236.88\ty=11032.97 \nLabel=Strip\t695\tX=885.21\ty=11089.43 \nLabel=Strip\t696\tX=1232.59\ty=11181.95 \nLabel=Strip\t697\tX=880.89\ty=11238.27 \nLabel=Strip\t698\tX=1228.24\ty=11330.93 \nLabel=Strip\t699\tX=876.52\ty=11387.11 \nLabel=Strip\t700\tX=1223.83\ty=11479.91 \nLabel=Strip\t701\tX=872.09\ty=11535.96 \nLabel=Strip\t702\tX=1219.36\ty=11628.88 \nLabel=Strip\t703\tX=867.60\ty=11684.80 \nLabel=Strip\t704\tX=1214.84\ty=11777.86 \nLabel=Strip\t705\tX=863.06\ty=11833.64 \nLabel=Strip\t706\tX=1210.26\ty=11926.83 \nLabel=Strip\t707\tX=858.45\ty=11982.48 \nLabel=Strip\t708\tX=1205.62\ty=12075.81 \nLabel=Strip\t709\tX=853.79\ty=12131.32 \nLabel=Strip\t710\tX=1200.92\ty=12224.78 \nLabel=Strip\t711\tX=849.07\ty=12280.16 \nLabel=Strip\t712\tX=1196.17\ty=12373.76 \nLabel=Strip\t713\tX=844.30\ty=12429.00 \nLabel=Strip\t714\tX=1191.35\ty=12522.73 \nLabel=Strip\t715\tX=839.46\ty=12577.83 \nLabel=Strip\t716\tX=1186.48\ty=12671.70 \nLabel=Strip\t717\tX=834.57\ty=12726.67 \nLabel=Strip\t718\tX=1181.56\ty=12820.68 \nLabel=Strip\t719\tX=829.62\ty=12875.51 \nLabel=Strip\t720\tX=1176.57\ty=12969.65 \nLabel=Strip\t721\tX=824.62\ty=13024.34 \nLabel=Strip\t722\tX=1171.53\ty=13118.62 \nLabel=Strip\t723\tX=819.55\ty=13173.18 \nLabel=Strip\t724\tX=1166.43\ty=13267.59 \nLabel=Strip\t725\tX=814.43\ty=13322.02 \nLabel=Strip\t726\tX=1161.27\ty=13416.56 \nLabel=Strip\t727\tX=809.25\ty=13470.85 \nLabel=Strip\t728\tX=1156.05\ty=13565.53 \nLabel=Strip\t729\tX=804.01\ty=13619.68 \nLabel=Strip\t730\tX=1150.78\ty=13714.50 \nLabel=Strip\t731\tX=798.72\ty=13768.52 \nLabel=Strip\t732\tX=1145.45\ty=13863.46 \nLabel=Strip\t733\tX=793.37\ty=13917.38 \nLabel=Strip\t734\tX=1140.06\ty=14012.43 \nLabel=Strip\t735\tX=787.96\ty=14066.18 \nLabel=Strip\t736\tX=1134.61\ty=14161.40 \nLabel=Strip\t737\tX=782.49\ty=14215.01 \nLabel=Strip\t738\tX=1129.11\ty=14310.36 \nLabel=Strip\t739\tX=776.97\ty=14363.84 \nLabel=Strip\t740\tX=1123.55\ty=14459.32 \nLabel=Strip\t741\tX=771.38\ty=14512.67 \nLabel=Strip\t742\tX=1117.93\ty=14608.29 \nLabel=Strip\t743\tX=765.74\ty=14661.50 \nLabel=Strip\t744\tX=1112.25\ty=14757.25 \nLabel=Strip\t745\tX=760.05\ty=14810.33 \nLabel=Strip\t746\tX=1106.51\ty=14906.21 \nLabel=Strip\t747\tX=754.29\ty=14959.15 \nLabel=Strip\t748\tX=1100.72\ty=15055.17 \nLabel=Strip\t749\tX=748.48\ty=15107.98 \nLabel=Strip\t750\tX=1094.87\ty=15204.13 \nLabel=Strip\t751\tX=742.61\ty=15256.80 \nLabel=Strip\t752\tX=1088.97\ty=15353.09 \nLabel=Strip\t753\tX=736.68\ty=15405.63 \nLabel=Strip\t754\tX=1083.00\ty=15502.05 \nLabel=Strip\t755\tX=730.69\ty=15554.45 \nLabel=Strip\t756\tX=1076.98\ty=15651.01 \nLabel=Strip\t757\tX=724.65\ty=15703.27 \nLabel=Strip\t758\tX=1070.90\ty=15799.96 \nLabel=Strip\t759\tX=718.55\ty=15852.09 \nLabel=Strip\t760\tX=1064.76\ty=15948.92 \nLabel=Strip\t761\tX=712.39\ty=16000.91 \nLabel=Strip\t762\tX=1058.56\ty=16097.87 \nLabel=Strip\t763\tX=706.17\ty=16149.73 \nLabel=Strip\t764\tX=1052.31\ty=16246.82 \nLabel=Strip\t765\tX=699.90\ty=16298.55 \nLabel=Strip\t766\tX=1046.00\ty=16395.78 \nLabel=Strip\t767\tX=693.57\ty=16447.36 \nLabel=Strip\t768\tX=1039.63\ty=16544.73 \nLabel=Strip\t769\tX=687.18\ty=16596.18 \nLabel=Strip\t770\tX=1033.20\ty=16693.68 \nLabel=Strip\t771\tX=680.73\ty=16744.99 \nLabel=Strip\t772\tX=1026.72\ty=16842.62 \nLabel=Strip\t773\tX=674.23\ty=16893.80 \nLabel=Strip\t774\tX=1020.18\ty=16991.57 \nLabel=Strip\t775\tX=667.67\ty=17042.61 \nLabel=Strip\t776\tX=1013.58\ty=17140.52 \nLabel=Strip\t777\tX=661.05\ty=17191.42 \nLabel=Strip\t778\tX=1006.92\ty=17289.46 \nLabel=Strip\t779\tX=654.37\ty=17340.23 \nLabel=Strip\t780\tX=1000.20\ty=17438.40 \nLabel=Strip\t781\tX=647.64\ty=17489.04 \nLabel=Strip\t782\tX=993.43\ty=17587.34 \nLabel=Strip\t783\tX=640.85\ty=17637.85 \nLabel=Strip\t784\tX=986.60\ty=17736.29 \nLabel=Strip\t785\tX=634.00\ty=17786.65 \nLabel=Strip\t786\tX=979.71\ty=17885.22 \nLabel=Strip\t787\tX=627.09\ty=17935.45 \nLabel=Strip\t788\tX=972.77\ty=18034.16 \nLabel=Strip\t789\tX=620.13\ty=18084.26 \nLabel=Strip\t790\tX=965.77\ty=18183.10 \nLabel=Strip\t791\tX=613.10\ty=18233.06 \nLabel=Strip\t792\tX=958.71\ty=18332.03 \nLabel=Strip\t793\tX=606.02\ty=18381.86 \nLabel=Strip\t794\tX=951.59\ty=18480.97 \nLabel=Strip\t795\tX=598.88\ty=18530.65 \nLabel=Strip\t796\tX=944.41\ty=18629.90 \nLabel=Strip\t797\tX=591.69\ty=18679.45 \nLabel=Strip\t798\tX=937.18\ty=18778.83 \nLabel=Strip\t799\tX=584.44\ty=18828.25 \nLabel=Strip\t800\tX=929.89\ty=18927.76 \nLabel=Strip\t801\tX=577.13\ty=18977.04 \nLabel=Strip\t802\tX=922.54\ty=19076.69 \nLabel=Strip\t803\tX=569.76\ty=19125.83 \nLabel=Strip\t804\tX=915.13\ty=19225.61 \nLabel=Strip\t805\tX=562.33\ty=19274.62 \nLabel=Strip\t806\tX=907.67\ty=19374.54 \nLabel=Strip\t807\tX=554.85\ty=19423.41 \nLabel=Strip\t808\tX=900.14\ty=19523.46 \nLabel=Strip\t809\tX=547.31\ty=19572.20 \nLabel=Strip\t810\tX=892.56\ty=19672.38 \nLabel=Strip\t811\tX=539.71\ty=19720.98 \nLabel=Strip\t812\tX=884.93\ty=19821.30 \nLabel=Strip\t813\tX=532.05\ty=19869.77 \nLabel=Strip\t814\tX=877.23\ty=19970.22 \nLabel=Strip\t815\tX=524.34\ty=20018.55 \nLabel=Strip\t816\tX=869.48\ty=20119.13 \nLabel=Strip\t817\tX=516.57\ty=20167.33 \nLabel=Strip\t818\tX=861.67\ty=20268.05 \nLabel=Strip\t819\tX=508.74\ty=20316.11 \nLabel=Strip\t820\tX=853.80\ty=20416.96 \nLabel=Strip\t821\tX=500.85\ty=20464.89 \nLabel=Strip\t822\tX=845.88\ty=20565.87 \nLabel=Strip\t823\tX=492.91\ty=20613.66 \nLabel=Strip\t824\tX=837.89\ty=20714.78 \nLabel=Strip\t825\tX=484.91\ty=20762.43 \nLabel=Strip\t826\tX=829.85\ty=20863.69 \nLabel=Strip\t827\tX=476.85\ty=20911.21 \nLabel=Strip\t828\tX=821.75\ty=21012.59 \nLabel=Strip\t829\tX=468.73\ty=21059.98 \nLabel=Strip\t830\tX=813.60\ty=21161.50 \nLabel=Strip\t831\tX=460.56\ty=21208.74 \nLabel=Strip\t832\tX=805.38\ty=21310.40 \nLabel=Strip\t833\tX=452.32\ty=21357.51 \nLabel=Strip\t834\tX=797.11\ty=21459.30 \nLabel=Strip\t835\tX=444.03\ty=21506.27 \nLabel=Strip\t836\tX=788.78\ty=21608.20 \nLabel=Strip\t837\tX=435.69\ty=21655.04 \nLabel=Strip\t838\tX=780.39\ty=21757.09 \nLabel=Strip\t839\tX=427.28\ty=21803.80 \nLabel=Strip\t840\tX=771.95\ty=21905.99 \nLabel=Strip\t841\tX=418.82\ty=21952.56 \nLabel=Strip\t842\tX=763.45\ty=22054.88 \nLabel=Strip\t843\tX=410.30\ty=22101.31 \nLabel=Strip\t844\tX=754.89\ty=22203.77 \nLabel=Strip\t845\tX=401.72\ty=22250.07 \nLabel=Strip\t846\tX=746.27\ty=22352.66 \nLabel=Strip\t847\tX=393.08\ty=22398.82 \nLabel=Strip\t848\tX=737.59\ty=22501.54 \nLabel=Strip\t849\tX=384.39\ty=22547.57 \nLabel=Strip\t850\tX=728.86\ty=22650.43 \nLabel=Strip\t851\tX=375.64\ty=22696.32 \nLabel=Strip\t852\tX=720.07\ty=22799.31 \nLabel=Strip\t853\tX=366.83\ty=22845.06 \nLabel=Strip\t854\tX=711.22\ty=22948.19 \nLabel=Strip\t855\tX=357.96\ty=22993.81 \nLabel=Strip\t856\tX=702.32\ty=23097.07 \nLabel=Strip\t857\tX=349.04\ty=23142.55 \nLabel=Strip\t858\tX=693.35\ty=23245.94 \nLabel=Strip\t859\tX=340.06\ty=23291.29 \nLabel=Strip\t860\tX=684.33\ty=23394.82 \nLabel=Strip\t861\tX=331.02\ty=23440.03 \nLabel=Strip\t862\tX=675.25\ty=23543.69 \nLabel=Strip\t863\tX=321.92\ty=23588.76 \nLabel=Strip\t864\tX=666.12\ty=23692.56 \nLabel=Strip\t865\tX=312.77\ty=23737.50 \nLabel=Strip\t866\tX=656.92\ty=23841.42 \nLabel=Strip\t867\tX=303.56\ty=23886.23 \nLabel=Strip\t868\tX=647.67\ty=23990.29 \nLabel=Strip\t869\tX=294.29\ty=24034.96 \nLabel=Strip\t870\tX=638.36\ty=24139.15 \nLabel=Strip\t871\tX=284.96\ty=24183.68 \nLabel=Strip\t872\tX=628.99\ty=24288.01 \nLabel=Strip\t873\tX=275.58\ty=24332.41 \nLabel=Strip\t874\tX=619.57\ty=24436.87 \nLabel=Strip\t875\tX=266.14\ty=24481.13 \nLabel=Strip\t876\tX=610.08\ty=24585.72 \nLabel=Strip\t877\tX=256.64\ty=24629.85 \nLabel=Strip\t878\tX=600.54\ty=24734.58 \nLabel=Strip\t879\tX=247.08\ty=24778.56 \nLabel=Strip\t880\tX=590.95\ty=24883.43 \nLabel=Strip\t881\tX=237.46\ty=24927.28 \nLabel=Strip\t882\tX=581.29\ty=25032.27 \nLabel=Strip\t883\tX=227.79\ty=25075.99 \nLabel=Strip\t884\tX=571.58\ty=25181.12 \nLabel=Strip\t885\tX=218.06\ty=25224.70 \nLabel=Strip\t886\tX=561.81\ty=25329.96 \nLabel=Strip\t887\tX=208.27\ty=25373.41 \nLabel=Strip\t888\tX=551.98\ty=25478.80 \nLabel=Strip\t889\tX=198.43\ty=25522.11 \nLabel=Strip\t890\tX=542.09\ty=25627.64 \nLabel=Strip\t891\tX=188.52\ty=25670.82 \nLabel=Strip\t892\tX=532.15\ty=25776.48 \nLabel=Strip\t893\tX=178.56\ty=25819.51 \nLabel=Strip\t894\tX=522.14\ty=25925.32 \nLabel=Strip\t895\tX=168.54\ty=25968.21 \nLabel=Strip\t896\tX=512.09\ty=26074.14 \nLabel=Strip\t897\tX=158.47\ty=26116.91 \nLabel=Strip\t898\tX=501.97\ty=26222.97 \nLabel=Strip\t899\tX=148.33\ty=26265.60 \nLabel=Strip\t900\tX=491.79\ty=26371.79 \nLabel=Strip\t901\tX=138.14\ty=26414.29 \nLabel=Strip\t902\tX=481.56\ty=26520.62 \nLabel=Strip\t903\tX=127.89\ty=26562.97 \nLabel=Strip\t904\tX=471.27\ty=26669.44 \nLabel=Strip\t905\tX=117.59\ty=26711.66 \nLabel=Strip\t906\tX=460.92\ty=26818.25 \nLabel=Strip\t907\tX=107.22\ty=26860.34 \nLabel=Strip\t908\tX=450.52\ty=26967.07 \nLabel=Strip\t909\tX=96.80\ty=27009.02 \nLabel=Strip\t910\tX=440.05\ty=27115.88 \nLabel=Strip\t911\tX=86.32\ty=27157.69 \nLabel=Strip\t912\tX=429.53\ty=27264.69 \nLabel=Strip\t913\tX=75.78\ty=27306.37 \nLabel=Strip\t914\tX=418.95\ty=27413.49 \nLabel=Strip\t915\tX=65.19\ty=27455.04 \nLabel=Strip\t916\tX=408.32\ty=27562.30 \nLabel=Strip\t917\tX=54.54\ty=27603.70 \nLabel=Strip\t918\tX=397.63\ty=27711.10 \nLabel=Strip\t919\tX=43.83\ty=27752.37 \nLabel=Strip\t920\tX=386.87\ty=27859.90 \nLabel=Strip\t921\tX=33.06\ty=27901.03 \nLabel=Strip\t922\tX=376.06\ty=28008.69 \nLabel=Strip\t923\tX=22.24\ty=28049.69 \nLabel=Strip\t924\tX=365.20\ty=28157.48 \nLabel=Strip\t925\tX=11.35\ty=28198.35 \nLabel=Strip\t926\tX=354.27\ty=28306.27 \nLabel=Strip\t927\tX=0.41\ty=28347.00 \nLabel=Strip\t928\tX=343.29\ty=28455.06 \nLabel=Strip\t929\tX=-10.59\ty=28495.65 \nLabel=Strip\t930\tX=332.25\ty=28603.84 \nLabel=Strip\t931\tX=-21.64\ty=28644.30 \nLabel=Strip\t932\tX=321.15\ty=28752.62 \nLabel=Strip\t933\tX=-32.75\ty=28792.94 \nLabel=Strip\t934\tX=310.00\ty=28901.40 \nLabel=Strip\t935\tX=-43.93\ty=28941.58 \nLabel=Strip\t936\tX=298.79\ty=29050.17 \nLabel=Strip\t937\tX=-55.15\ty=29090.22 \nLabel=Strip\t938\tX=287.52\ty=29198.94 \nLabel=Strip\t939\tX=-66.44\ty=29238.85 \nLabel=Strip\t940\tX=276.19\ty=29347.71 \nLabel=Strip\t941\tX=-77.78\ty=29387.49 \nLabel=Strip\t942\tX=264.80\ty=29496.48 \nLabel=Strip\t943\tX=-89.18\ty=29536.11 \nLabel=Strip\t944\tX=253.36\ty=29645.24 \nLabel=Strip\t945\tX=-100.64\ty=29684.74 \nLabel=Strip\t946\tX=241.86\ty=29794.00 \nLabel=Strip\t947\tX=-112.16\ty=29833.36 \nLabel=Strip\t948\tX=230.30\ty=29942.75 \nLabel=Strip\t949\tX=-123.73\ty=29981.98 \nLabel=Strip\t950\tX=218.68\ty=30091.50 \nLabel=Strip\t951\tX=-135.37\ty=30130.60 \nLabel=Strip\t952\tX=207.01\ty=30240.25 \nLabel=Strip\t953\tX=-147.06\ty=30279.21 \nLabel=Strip\t954\tX=195.28\ty=30389.00 \nLabel=Strip\t955\tX=-158.80\ty=30427.82 \nLabel=Strip\t956\tX=183.49\ty=30537.74 \nLabel=Strip\t957\tX=-170.61\ty=30576.43 \nLabel=Strip\t958\tX=171.64\ty=30686.48 \nLabel=Strip\t959\tX=-182.47\ty=30725.03 \nLabel=Strip\t960\tX=159.73\ty=30835.22 \nLabel=Strip\t
